vi "Test Display_LE.vi"(0 "LEUI_LEDs_Actual":T1, 1 "LEUI_LEDs_Expected":T1, 2 "Care":T1, 11 "Error In":errorcluster) -> (4 "Pass/Fail?":bool, 6 "Report Text":string, 15 "Error Out":errorcluster)   [LabVIEW 2016, in "TL27.lvlib"]
uses:
  Projects/TL27.lvlib
  controls/LEUI_LEDs.ctl
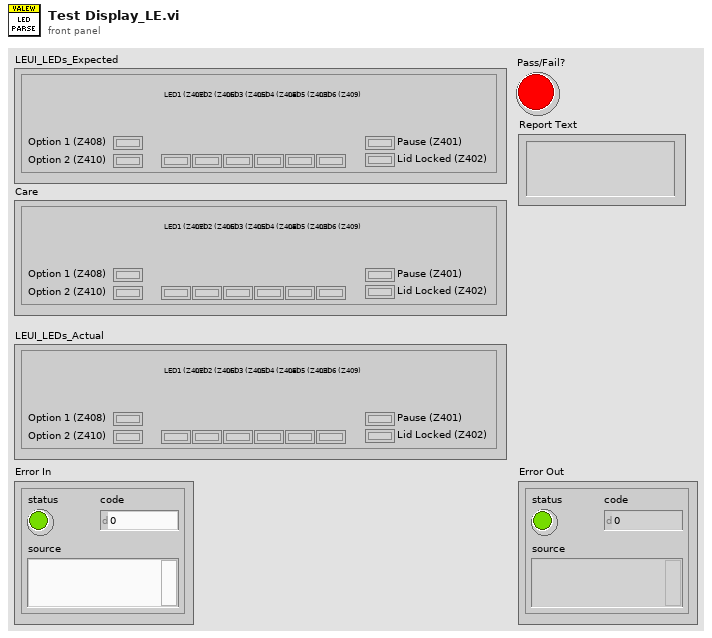
[diagram p1: front panel]
types:
  T1 = typedef "TL27.lvlib/LEUI_LEDs.ctl" = cluster{"Pause (Z401)":bool, "Lid Locked (Z402)":bool, "LED1 (Z407)":bool, "LED2 (Z406)":bool, "LED3 (Z405)":bool, "LED4 (Z404)":bool, "LED5 (Z403)":bool, "LED6 (Z409)":bool, "Option 1 (Z408)":bool, "Option 2 (Z410)":bool}
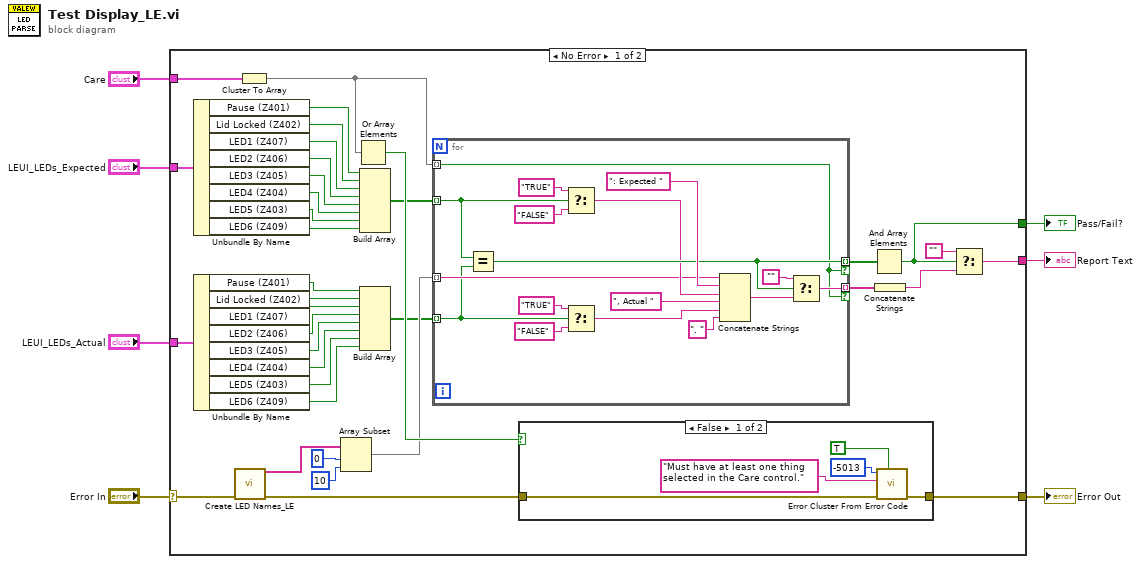
[diagram p0: block diagram]
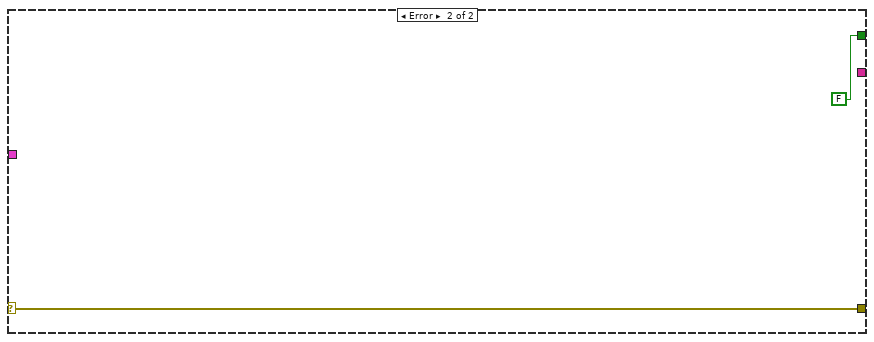
[diagram p3: hidden frame]
diagram:
  n1 = case shown="No Error" "Error In" {
    selector: "Error In" -> [w41 w68]
    tunnel: [w25 w68] -> w5
    tunnel: [w42 _] -> w7
    tunnel: "Care" -> [w39 _]
    tunnel: "LEUI_LEDs_Expected" -> [w9 _]
    tunnel: "LEUI_LEDs_Actual" -> [w12 _]
    tunnel: [w10 FALSE] -> w6
    frame No Error {
      n2 = Unbundle By Name(w9) -> ("Pause (Z401)"=w29:bool, "Lid Locked (Z402)"=w28:bool, "LED1 (Z407)"=w27:bool, "LED2 (Z406)"=w26:bool, "LED3 (Z405)"=w24:bool, "LED4 (Z404)"=w23:bool, "LED5 (Z403)"=w22:bool, "LED6 (Z409)"=w21:bool)
      n3 = Unbundle By Name(w12) -> ("Pause (Z401)"=w20:bool, "Lid Locked (Z402)"=w19:bool, "LED1 (Z407)"=w18:bool, "LED2 (Z406)"=w17:bool, "LED3 (Z405)"=w16:bool, "LED4 (Z404)"=w15:bool, "LED5 (Z403)"=w14:bool, "LED6 (Z409)"=w13:bool)
      n4 = call "Create LED Names_LE.vi"("Error In"=w41) -> ("Names"=w33:string[], "Error Out"=w38:errorcluster)  [unwired: 13 in]
      n5 = Cluster To Array(cluster=w39) -> (array=w8:bool[])
      n6 = Array Subset(array=w33, index=0, length=10) -> (w34:string[])
      n7 = Or Array Elements(Boolean array=w8) -> (logical OR=w40:bool)
      n8 = Build Array(w29, w28, w27, w26, w24, w23, w22, w21) -> (w37:bool[])
      n9 = Build Array(w20, w19, w18, w17, w16, w15, w14, w13) -> (w11:bool[])
      n10 = for {
        tunnel: w11 -> [w44] mode=indexing
        tunnel: w37 -> [w45] mode=indexing
        tunnel: [w55] -> w32 mode=indexing if=w53
        tunnel: [w54] -> w30 mode=indexing if=w53
        tunnel: w8 -> [w53] mode=indexing
        tunnel: w34 -> [w46] mode=indexing
        n11 = Equal?(x=w45, y=w44) -> (x = y?=w54:bool)
        n12 = Select(t="TRUE" ("string"), s=w45, f="FALSE" ("string")) -> (s? t:f=w47:string)
        n13 = Select(t="TRUE" ("string"), s=w44, f="FALSE" ("string")) -> (s? t:f=w50:string)
        n14 = Concatenate Strings(w46, ": Expected " ("string"), w47, ", Actual " ("string"), w50, ". " ("string")) -> (w56:string)
        n15 = Select(t="", s=w54, f=w56) -> (s? t:f=w55:string)
      }
      n16 = case shown="False" w40 {
        tunnel: w38 -> [w65 w66]
        tunnel: [w64 w66] -> w25
        frame False {
          n17 = call <vilib>:"Error Cluster From Error Code.vi"("show call chain? (False)"=TRUE, "error in (no error)"=w65, "error message (\"\")"="Must have at least one thing selected in the Care control." ("error message (\"\")"), "error code (0)"=-5013) -> ("error out"=w64:errorcluster)  [unwired: 5 in]
        }
        frame True {
        }
      }
      n18 = And Array Elements(Boolean array=w30) -> (logical AND=w10:bool)
      n19 = Concatenate Strings(w32) -> (w31:string)
      n20 = Select(t="", s=w10, f=w31) -> (s? t:f=w42:string)
    }
    frame Error {
    }
  }
  "Report Text" <- w7
  "Pass/Fail?" <- w6
  "Error Out" <- w5
